vi "Read Attributes.vi"(11 "Return Setpoint Msg":refnum<class "Return Setpoint Msg.lvclass">) -> (2 "Payload":cluster{"DeviceID":u64, "Setpoints":dbl[]})   [LabVIEW 2016, in "Optimization Framework.lvlib" / "Return Setpoint Msg.lvclass"]
uses:
  Return Setpoint Msg.lvclass
  Return Setpoint Msg.lvclass/Return Setpoint Msg.ctl
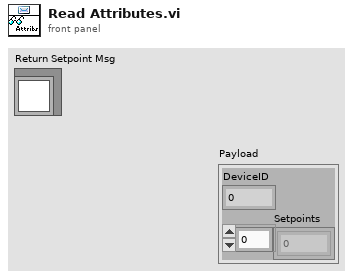
[diagram p1: front panel]
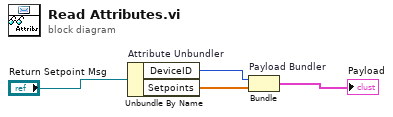
[diagram p0: block diagram]
diagram:
  n1 = Unbundle By Name "Attribute Unbundler"("Return Setpoint Msg") -> ("DeviceID"=w1:u64, "Setpoints"=w2:dbl[])
  n2 = Bundle "Payload Bundler"("DeviceID"=w1, "Setpoints"=w2) -> (→"Payload":cluster{"DeviceID":u64, "Setpoints":dbl[]})  [unwired: 1 in]
